vi "TeleopControls.vi"() -> ()   [LabVIEW 2018]
uses:
  <vilib>/Rock Robotics/WPI/ThirdParty/Phoenix-LabVIEW/Motor Controller/Controls/CTRE_Phoenix_MotorControl_ControlMode.ctl
  <vilib>/Rock Robotics/WPI/Relay/WPI_RelayValue.ctl
  <vilib>/Rock Robotics/WPI/Utilities/WPI_GetSetVariantRefNum.vi
  <vilib>/Rock Robotics/WPI/ThirdParty/Phoenix-LabVIEW/Motor Controller/Get/CTRE_Phoenix_MotorController_GetLimitSwitchStates.vi
  Swerve/SwerveGlobals.vi
panel:
  in  "AutoClimb":bool
  # "Copilot controls:\nRight button: set arm out\nRight switch: hold down to release hatch from hatch catch\nLeft button: set arm in\nLeft switch: Cargo out?\nA button: lift low\nB button: lift mid\nY button: lift high\nRight joystick button: Start automated climb sequence\nRight joystick y axis: Up/down all climb actuators\nLeft joystick y axis: Move forward climbing\nPOV hat right: Up front climb actuator\nPOV hat left: Up back climb actuators"
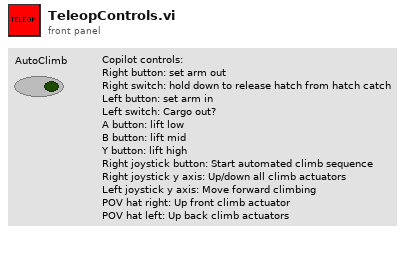
[diagram p1: front panel]
types:
  T1 = typedef "WPI_JoystickDevRef.ctl" = cluster{"Device":T2}
  T2 = typedef "WPI_JoystickDeviceEnum.ctl" = enum16{"USB 0", "USB 1", "USB 2", "USB 3", "USB 4", "USB 5"}
  T3 = typedef "WPI_RelayDevRef.ctl" = cluster{"DevStatus":errorcluster, "Relay Channel":T4, "Relay Direction":T5}
  T4 = typedef "FPGA_DIORelayChannel.ctl" = enum8{"Relay 0", "Relay 1", "Relay 2", "Relay 3", "Invalid"}
  T5 = typedef "WPI_RelayDirection.ctl" = enum16{"Both directions", "Forward only", "Reverse only"}
  T6 = typedef "WPI_MotorControlDeviceRef.ctl" = cluster{"DeviceStatus":errorcluster, "Type":T7, "PWM":cluster{"PWM Channel":T8, "DeadBand":T9}, "CAN":cluster{"Device Number":u8, "SetOutput VI Ref":variant, "GetOutput VI Ref":variant, "Enable VI Ref":variant, "Disable VI Ref":variant, "Data":variant}, "Invert":bool, "DIO PWM":cluster{"PWM \"Enable\" Channel":T8, "DIOChannel":T10, "PWM Rate":dbl}}
  T7 = typedef "WPI_MotorControlType.ctl" = enum16{"PWM", "CAN", "DIO PWM"}
  T8 = typedef "FPGA_DIOPWMChannel.ctl" = enum8{"PWM 0", "PWM 1", "PWM 2", "PWM 3", "PWM 4", "PWM 5", "PWM 6", "PWM 7", "PWM 8", "PWM 9", "PWM MXP 0", "PWM MXP 1", "PWM MXP 2", "PWM MXP 3", "PWM MXP 4", "PWM MXP 5", "PWM MXP 6", "PWM MXP 7", "PWM MXP 8", "PWM MXP 9", "Invalid"}
  T9 = typedef "WPI_PWMDeadband.ctl" = cluster{"Name":string, "maxPositivePwm":i32, "minPositivePwm":i32, "centerPwm":i32, "maxNegativePwm":i32, "minNegativePwm":i32, "angularRange":u16}
  T10 = typedef "FPGA_DIOChannel.ctl" = enum8{"DIO 0", "DIO 1", "DIO 2", "DIO 3", "DIO 4", "DIO 5", "DIO 6", "DIO 7", "DIO 8", "DIO 9", "DIO MXP 0", "DIO MXP 1", "DIO MXP 2", "DIO MXP 3", "DIO MXP 4", "DIO MXP 5", "DIO MXP 6", "DIO MXP 7", "DIO MXP 8", "DIO MXP 9", "DIO MXP 10", "DIO MXP 11", "DIO MXP 12", "DIO MXP 13", "DIO MXP 14", "DIO MXP 15", "SPI Port CS1", "SPI Port CS2", "SPI Port CS3", "SPI Port MISO", "SPI Port MOSI", "Invalid"}
  T11 = typedef "WPI_EncoderDevRef.ctl" = cluster{"DevStatus":errorcluster, "EncoderIndex":T12, "CounterIndex":T13, "DistancePerCount":dbl, "Decoding Type":T14}
  T12 = typedef "FPGA_EncoderIdx.ctl" = enum8{"Enc 0", "Enc 1", "Enc 2", "Enc 3", "Enc 4", "Enc 5", "Enc 6", "Enc 7", "Invalid"}
  T13 = typedef "FPGA_CounterCtrSystemIndex.ctl" = enum8{"Ctr 0", "Ctr 1", "Ctr 2", "Ctr 3", "Ctr 4", "Ctr 5", "Ctr 6", "Ctr 7", "Invalid"}
  T14 = typedef "WPI_EncoderType.ctl" = enum16{"1x", "2x", "4x"}
  T15 = typedef "WPI_RelayValue.ctl" = enum16{"Off", "On", "Forward", "Reverse"}
  T16 = typedef "CTRE_Phoenix_MotorControl_ControlMode.ctl" = u16
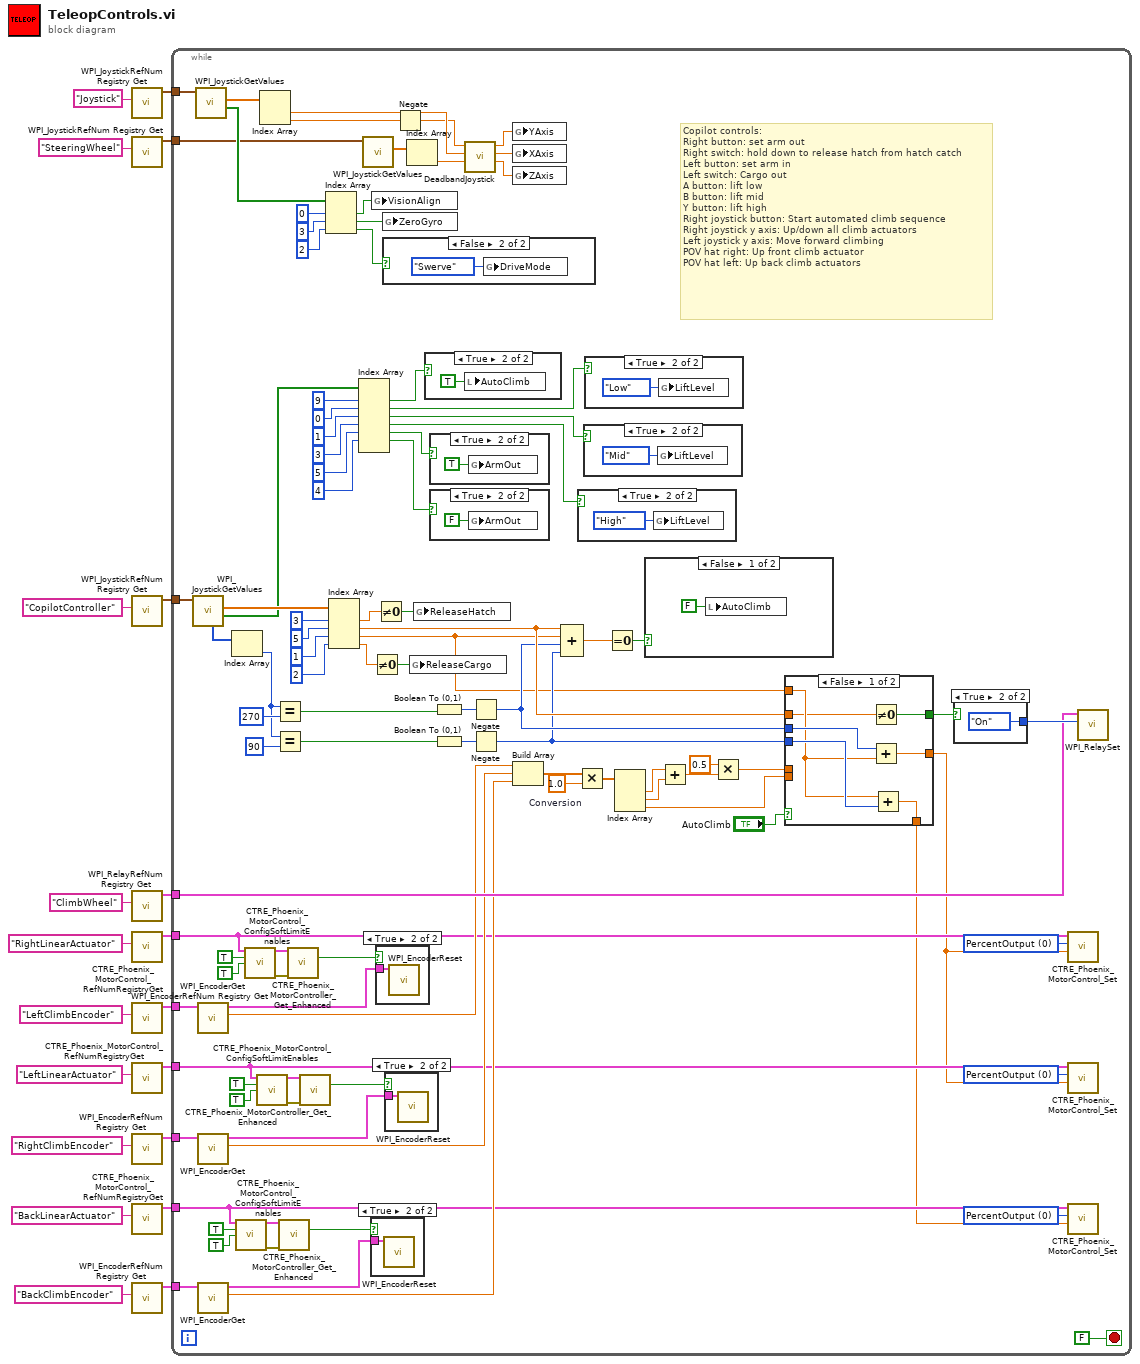
[diagram p0: block diagram]
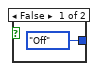
[diagram p5: hidden frame]
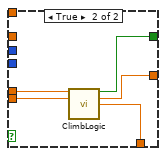
[diagram p12: hidden frame]
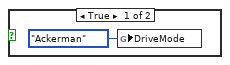
[diagram p14: hidden frame]
diagram:
  n1 = call <vilib>:"WPI_JoystickRefNum Registry Get.vi"("refnum name"="Joystick") -> ("JoystickDevRef"=w17:T1)  [unwired: 1 in, 9 out]
  n2 = call <vilib>:"WPI_JoystickRefNum Registry Get.vi"("refnum name"="SteeringWheel") -> ("JoystickDevRef"=w16:T1)  [unwired: 1 in, 9 out]
  n3 = call <vilib>:"WPI_JoystickRefNum Registry Get.vi"("refnum name"="CopilotController") -> ("JoystickDevRef"=w15:T1)  [unwired: 1 in, 9 out]
  n4 = call <vilib>:"WPI_RelayRefNum Registry Get.vi"("refnum name"="ClimbWheel") -> ("RelayDevRef"=w13:T3)  [unwired: 9 in, 1 out]
  n5 = call <vilib>:"CTRE_Phoenix_MotorControl_RefNumRegistryGet.vi"("refnum name"="RightLinearActuator") -> ("PhoenixMotorControlDevRef"=w5:T6)  [unwired: 9 in, 1 out]
  n6 = call <vilib>:"WPI_EncoderRefNum Registry Get.vi"("refnum name"="LeftClimbEncoder") -> ("EncoderDevRef"=w9:T11)  [unwired: 9 in, 1 out]
  n7 = call <vilib>:"CTRE_Phoenix_MotorControl_RefNumRegistryGet.vi"("refnum name"="LeftLinearActuator") -> ("PhoenixMotorControlDevRef"=w4:T6)  [unwired: 9 in, 1 out]
  n8 = call <vilib>:"WPI_EncoderRefNum Registry Get.vi"("refnum name"="RightClimbEncoder") -> ("EncoderDevRef"=w8:T11)  [unwired: 9 in, 1 out]
  n9 = call <vilib>:"CTRE_Phoenix_MotorControl_RefNumRegistryGet.vi"("refnum name"="BackLinearActuator") -> ("PhoenixMotorControlDevRef"=w1:T6)  [unwired: 9 in, 1 out]
  n10 = call <vilib>:"WPI_EncoderRefNum Registry Get.vi"("refnum name"="BackClimbEncoder") -> ("EncoderDevRef"=w7:T11)  [unwired: 9 in, 1 out]
  n11 = while {
    tunnel: w17 -> [w86]
    tunnel: w16 -> [w85]
    tunnel: w15 -> [w84]
    tunnel: w13 -> [w68]
    tunnel: w5 -> [w33]
    tunnel: w4 -> [w34]
    tunnel: w1 -> [w27]
    tunnel: w9 -> [w56]
    tunnel: w8 -> [w55]
    tunnel: w7 -> [w54]
    stop <- FALSE stop-if-true
    w48 = T16 0 items=["PercentOutput"=0, "Position"=1, "Velocity"=2, "Current"=3, "Follower"=5, "MotionProfile"=6, "MotionMagic"=7, "MotionProfileArc"=10, "Disabled"=15] ("Control Mode")
    w49 = T16 0 items=["PercentOutput"=0, "Position"=1, "Velocity"=2, "Current"=3, "Follower"=5, "MotionProfile"=6, "MotionMagic"=7, "MotionProfileArc"=10, "Disabled"=15] ("Control Mode")
    w50 = T16 0 items=["PercentOutput"=0, "Position"=1, "Velocity"=2, "Current"=3, "Follower"=5, "MotionProfile"=6, "MotionMagic"=7, "MotionProfileArc"=10, "Disabled"=15] ("Control Mode")
    w58 = 1.0  # Conversion
    # "Copilot controls:\nRight button: set arm out\nRight switch: hold down to release hatch from hatch catch\nLeft button: set arm in\nLeft switch: Cargo out\nA button: lift low\nB button: lift mid\nY button: lift high\nRight joystick button: Start automated climb sequence\nRight joystick y axis: Up/down all climb actuators\nLeft joystick y axis: Move forward climbing\nPOV hat right: Up front climb actuator\nPOV hat left: Up back climb actuators"
    n12 = call <vilib>:"WPI_JoystickGetValues.vi"("JoystickDevRef"=w84) -> ("Buttons"=w71:bool[], "Axes"=w106:dbl[], "POVs"=w97:i16[])  [unwired: 6 in, 2 out]
    n13 = call <vilib>:"WPI_JoystickGetValues.vi"("JoystickDevRef"=w86) -> ("Buttons"=w118:bool[], "Axes"=w120:dbl[])  [unwired: 6 in, 3 out]
    n14 = call <vilib>:"WPI_EncoderGet.vi"("EncoderDevRef"=w56) -> ("Distance"=w66:dbl, "EncoderDevRef"=w45:T11)  [unwired: 5 in, 4 out]
    n15 = call <vilib>:"WPI_EncoderGet.vi"("EncoderDevRef"=w55) -> ("Distance"=w65:dbl, "EncoderDevRef"=w43:T11)  [unwired: 5 in, 4 out]
    n16 = call <vilib>:"WPI_EncoderGet.vi"("EncoderDevRef"=w54) -> ("Distance"=w64:dbl, "EncoderDevRef"=w42:T11)  [unwired: 5 in, 4 out]
    n17 = Index Array(array=w97) -> (element=w94:i16)  [unwired: 1 in]
    n18 = call <vilib>:"CTRE_Phoenix_MotorControl_ConfigSoftLimitEnables.vi"("PhoenixMotorControlDevRef"=w27, "Forward Soft Limit Enable"=TRUE, "Reverse Soft Limit Enable"=TRUE) -> ("PhoenixMotorControlDevRef"=w32:T6, "error out"=w31:errorcluster)  [unwired: 11 in]
    n19 = call <vilib>:"CTRE_Phoenix_MotorControl_ConfigSoftLimitEnables.vi"("PhoenixMotorControlDevRef"=w33, "Forward Soft Limit Enable"=TRUE, "Reverse Soft Limit Enable"=TRUE) -> ("PhoenixMotorControlDevRef"=w47:T6, "error out"=w46:errorcluster)  [unwired: 11 in]
    n20 = call <vilib>:"CTRE_Phoenix_MotorControl_ConfigSoftLimitEnables.vi"("PhoenixMotorControlDevRef"=w34, "Forward Soft Limit Enable"=TRUE, "Reverse Soft Limit Enable"=TRUE) -> ("PhoenixMotorControlDevRef"=w39:T6, "error out"=w38:errorcluster)  [unwired: 11 in]
    n21 = Index Array(array=w120) -> (element #1=w108:dbl, element #2=w119:dbl)  [unwired: 2 in]
    n22 = Equal?(x=w94, y=i16 270) -> (x = y?=w89:bool)
    n23 = Equal?(x=w94, y=i16 90) -> (x = y?=w88:bool)
    n24 = call-poly <vilib>:"CTRE_Phoenix_MotorController_Get_Enhanced.vi"("PhoenixMotorControlDevRef"=w32, "error in"=w31) -> ("Forward Limit Closed?"=w28:bool)  [unwired: 10 in, 3 out]
    n25 = call-poly <vilib>:"CTRE_Phoenix_MotorController_Get_Enhanced.vi"("PhoenixMotorControlDevRef"=w47, "error in"=w46) -> ("Forward Limit Closed?"=w44:bool)  [unwired: 10 in, 3 out]
    n26 = call-poly <vilib>:"CTRE_Phoenix_MotorController_Get_Enhanced.vi"("PhoenixMotorControlDevRef"=w39, "error in"=w38) -> ("Forward Limit Closed?"=w35:bool)  [unwired: 10 in, 3 out]
    n27 = Index Array(array=w118, index #1=0 ("index"), index #2=3 ("index"), index #3=2 ("index")) -> (element #1=w114:bool, element #2=w101:bool, element #3=w115:bool)
    n28 = Index Array(array=w106, index #1=3 ("index"), index #2=5 ("index"), index #3=1 ("index"), index #4=2 ("index")) -> (element #1=w107:dbl, element #2=w99:dbl, element #3=w24:dbl, element #4=w21:dbl)
    n29 = Index Array(array=w71, index #1=9 ("index"), index #2=0 ("index"), index #3=1 ("index"), index #4=3 ("index"), index #5=5 ("index"), index #6=4 ("index")) -> (element #1=w77:bool, element #2=w74:bool, element #3=w76:bool, element #4=w75:bool, element #5=w72:bool, element #6=w73:bool)  [unwired: 1 in, 1 out]
    n30 = call <vilib>:"WPI_JoystickGetValues.vi"("JoystickDevRef"=w85) -> ("Axes"=w121:dbl[])  [unwired: 6 in, 4 out]
    n31 = case shown="True" w28 {
      tunnel: w42 -> [_ w122]
      frame False {
      }
      frame True {
        n32 = call <vilib>:"WPI_EncoderReset.vi"("EncoderDevRef"=w122) -> ()  [unwired: 9 in, 2 out]
      }
    }
    n33 = global write "SwerveGlobals.vi" "VisionAlign"(w114) -> ()
    n34 = Not Equal To 0?(x=w21) -> (x != 0?=w22:bool)
    n35 = Not Equal To 0?(x=w107) -> (x != 0?=w100:bool)
    n36 = case shown="True" w44 {
      tunnel: w45 -> [_ w124]
      frame False {
      }
      frame True {
        n37 = call <vilib>:"WPI_EncoderReset.vi"("EncoderDevRef"=w124) -> ()  [unwired: 9 in, 2 out]
      }
    }
    n38 = global write "SwerveGlobals.vi" "ZeroGyro"(w101) -> ()
    n39 = case shown="False" w115 {
      frame True {
        n40 = global write "SwerveGlobals.vi" "DriveMode"(enum16{"Swerve", "Ackerman"}."Ackerman" ("DriveMode")) -> ()
      }
      frame False {
        n41 = global write "SwerveGlobals.vi" "DriveMode"(enum16{"Swerve", "Ackerman"}."Swerve" ("DriveMode")) -> ()
      }
    }
    n42 = case shown="True" w35 {
      tunnel: w43 -> [_ w123]
      frame False {
      }
      frame True {
        n43 = call <vilib>:"WPI_EncoderReset.vi"("EncoderDevRef"=w123) -> ()  [unwired: 9 in, 2 out]
      }
    }
    n44 = Negate(x=w119) -> (-x=w102:dbl)
    n45 = Index Array(array=w121) -> (element=w109:dbl)  [unwired: 1 in]
    n46 = global write "SwerveGlobals.vi" "ReleaseCargo"(w22) -> ()
    n47 = global write "SwerveGlobals.vi" "ReleaseHatch"(w100) -> ()
    n48 = case shown="True" w77 {
      frame False {
      }
      frame True {
        n49 = local write "AutoClimb"(TRUE ("AutoClimb")) -> ()
      }
    }
    n50 = case shown="True" w72 {
      frame False {
      }
      frame True {
        n51 = global write "SwerveGlobals.vi" "ArmOut"(TRUE ("ArmOut")) -> ()
      }
    }
    n52 = case shown="True" w73 {
      frame False {
      }
      frame True {
        n53 = global write "SwerveGlobals.vi" "ArmOut"(FALSE ("ArmOut")) -> ()
      }
    }
    n54 = Boolean To (0,1)(Boolean=w89) -> (0, 1=w90:i16)
    n55 = Boolean To (0,1)(Boolean=w88) -> (0, 1=w91:i16)
    n56 = call "DeadbandJoystick.vi"("Z"=w109, "Y"=w108, "X"=w102) -> ("Z'"=w110:dbl, "Y'"=w112:dbl, "X'"=w111:dbl)  [unwired: 6 in]
    n57 = Negate(x=w90) -> (-x=w87:i16)
    n58 = Negate(x=w91) -> (-x=w53:i16)
    n59 = global write "SwerveGlobals.vi" "YAxis"(w111) -> ()
    n60 = global write "SwerveGlobals.vi" "XAxis"(w112) -> ()
    n61 = global write "SwerveGlobals.vi" "ZAxis"(w110) -> ()
    n62 = Build Array(w66, w65, w64) -> (w63:dbl[])
    n63 = Compound Arithmetic op=ADD(w99, w24, w87, w53) -> (w93:dbl)
    n64 = Multiply(x=w63, y=w58) -> (x*y=w62:dbl[])
    n65 = case shown="True" w75 {
      frame False {
      }
      frame True {
        n66 = global write "SwerveGlobals.vi" "LiftLevel"(enum16{"Low", "Mid", "High"}."High" ("LiftLevel")) -> ()
      }
    }
    n67 = case shown="True" w76 {
      frame False {
      }
      frame True {
        n68 = global write "SwerveGlobals.vi" "LiftLevel"(enum16{"Low", "Mid", "High"}."Mid" ("LiftLevel")) -> ()
      }
    }
    n69 = case shown="True" w74 {
      frame False {
      }
      frame True {
        n70 = global write "SwerveGlobals.vi" "LiftLevel"(enum16{"Low", "Mid", "High"}."Low" ("LiftLevel")) -> ()
      }
    }
    n71 = Equal To 0?(x=w93) -> (x = 0?=w98:bool)
    n72 = Index Array(array=w62) -> (element #1=w61:dbl, element #2=w60:dbl, element #3=w51:dbl)  [unwired: 3 in]
    n73 = case shown="False" w98 {
      frame False {
        n74 = local write "AutoClimb"(FALSE ("AutoClimb")) -> ()
      }
      frame True {
      }
    }
    n75 = Add(x=w61, y=w60) -> (x+y=w59:dbl)
    n76 = Multiply(x=0.5, y=w59) -> (x*y=w52:dbl)
    n77 = case shown="False" "AutoClimb" {
      tunnel: [w138 w144] -> w25
      tunnel: [w134 w143] -> w69
      tunnel: w99 -> [w135 _]
      tunnel: w87 -> [w139 _]
      tunnel: w53 -> [w137 _]
      tunnel: w24 -> [w136 _]
      tunnel: w52 -> [_ w142]
      tunnel: w51 -> [_ w141]
      tunnel: [w133 w140] -> w26
      frame False {
        n78 = Not Equal To 0?(x=w135) -> (x != 0?=w134:bool)
        n79 = Add(x=w139, y=w136) -> (x+y=w138:dbl)
        n80 = Add(x=w136, y=w137) -> (x+y=w133:dbl)
      }
      frame True {
        n81 = call "ClimbLogic.vi"("FrontClimbEncoder"=w142, "BackClimbEncoder"=w141) -> ("ClimbDrive"=w143:bool, "ActuateFrontClimb"=w144:dbl, "ActuateBackClimb"=w140:dbl)  [unwired: 11 in]
      }
    }
    n82 = case shown="True" w69 {
      tunnel: [WPI_RelayValue."Off" ("RelayValue") WPI_RelayValue."On" ("RelayValue")] -> w70
      frame False {
      }
      frame True {
      }
    }
    n83 = call <vilib>:"CTRE_Phoenix_MotorControl_Set.vi"("Output"=w25, "Control Mode"=w50, "PhoenixMotorControlDevRef"=w33) -> ()  [unwired: 6 in, 3 out]
    n84 = call <vilib>:"CTRE_Phoenix_MotorControl_Set.vi"("Output"=w25, "Control Mode"=w49, "PhoenixMotorControlDevRef"=w34) -> ()  [unwired: 6 in, 3 out]
    n85 = call <vilib>:"CTRE_Phoenix_MotorControl_Set.vi"("Output"=w26, "Control Mode"=w48, "PhoenixMotorControlDevRef"=w27) -> ()  [unwired: 6 in, 3 out]
    n86 = call <vilib>:"WPI_RelaySet.vi"("RelayValue"=w70, "RelayDevRef"=w68) -> ()  [unwired: 8 in, 2 out]
  }
